vi "TDS - Eurotherm.vi"() -> ()   [LabVIEW 2020]
uses:
  Control 2.ctl
  <instrlib>/rga_lv_85/SRSRGA85.llb/SRSRGAo Units Enumeration.ctl
  <instrlib>/rga_lv_85/SRSRGA85.llb/SRSRGAo RefNum.ctl
  <vilib>/Utility/sysdir.llb/System Directory Type.ctl
  <vilib>/Waveform/WDTFileIO.llb/Export Waveforms To Spreadsheet File (1D).vi
  custom-labview-lib-customlibs/customlib.lvlib
panel:
  out "VISA class":refnum<visa-resource-name>
  out "Process Value":sgl format="%.3g"
  in  "Reference Tab":refnum<vi>[](array[refnum])
  out "heat_LastData":dbl[](array[numeric])
  in  "Reconnect":bool
  out "RGA_LastData":sgl[](array[numeric]) format="%.2f"
  out "size(s) 3":i32
  out "HEAT start time":timestamp=timestamp(3621395400.2120705 s since 1904-01-01)
  out "Label.Text":string="D"
  out "Array 2":waveform(dbl)[](array[waveform])
  out "RGA data":waveform(dbl)[](array[waveform])=[{"t0"=timestamp(3621395444.273366 s since 1904-01-01), "dt"=0.25, "Y"=[0.0]}]
  out "output array":sgl[][](array[numeric])=[[8.752041e-08, 0.0, 0.0, 0.0]]
  out "Boolean":T1=TRUE
  out "stopped_loops":bool=TRUE
  in  "Tab Control":enum32{"Main", "XY Graph", "RGA"}(tab)
  in  "Start 1":bool=TRUE
  in  "Clear ALL":bool
  out "Waveform Graph":waveform(dbl)[](graph)
  out "main Graph":T2(graph)
  in  "Start 3":bool=TRUE
  out "XY Graph 2":cluster{dbl[], dbl[]}[](graph)
  in  "START RGA":bool
  out "Loop Time [ms]":u32=251
  in  "stop 3":bool
  in  "Rate (sec)":dbl=0.25 min=0.001
  out "P vs. t":sgl[][](graph)=[[8.752041e-08, 0.0, 0.0, 0.0]]
  in  "Tab Control 2":enum32{"Eurotherm"}(tab)
  out "Process Value":dbl
  in  "Save Data As":bool
  in  "Tab Control 3":enum32{"RGA control", "RGA setting"}(tab)
  out "CEM:":bool
  out "Filament:":bool
  in  "Disconnect":bool
  in  "Connect":bool
  in  "Connection Type:":u16(ring)=1 items=["Ethernet", "Serial"]
  in  "Specifications":T3(array[cluster])=[{"Mass"=2, "Noise Floor"=4, "CEM "=FALSE}] {"Noise Floor" min=0 max=7; "Mass" min=1 max=100}
  in  "Units:":T4
  in  "CEM:":bool
  in  "Filament:":bool
  out "Conected:":bool
  out "Error:":bool
  in  "START RGA  2":bool
  in  "stop 4":bool
  in  "Electron Emission [mA]":sgl=1.0 format="%.2f"
  out "Act. Electron Emission":sgl format="%.2f"
  out "Numeric":i32
  out "error out":errorcluster
  in  "ionizer":bool
  in  "detector":bool
  in  "stop":bool=TRUE
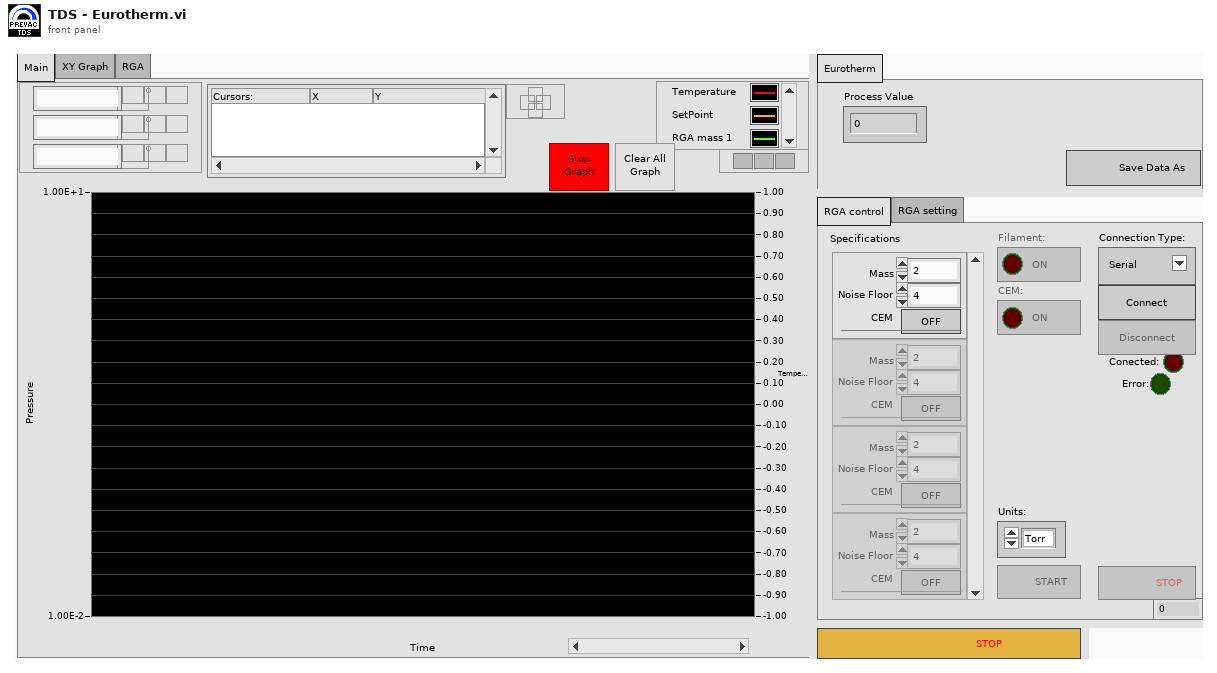
[diagram p1: front panel]
types:
  T1 = typedef "Control 2.ctl" = bool
  T2 = cluster{"heat_LastData[0]":dbl, "heat_LastData[1]":dbl, "heat_LastData[2]":dbl, "heat_LastData[3]":dbl, "heat_LastData[4]":dbl, "heat_LastData[5]":dbl, "heat_LastData[6]":dbl, "heat_LastData[7]":dbl, "heat_LastData[8]":dbl}
  T3 = cluster{"Mass":i32, "Noise Floor":i32, "CEM ":bool}[]
  T4 = typedef "SRSRGAo Units Enumeration.ctl" = enum16{"Torr", "mTorr", "mbar", "bar", "Pa", "A", "ppm"}
  T5 = typedef "SRSRGAo RefNum.ctl" = u16
  T6 = cluster{"heat_LastData[0]":dbl, "heat_LastData[1]":dbl, "heat_LastData[2]":dbl, "heat_LastData[3]":dbl, "heat_LastData[4]":dbl, "heat_LastData[5]":dbl, "heat_LastData[6]":dbl, "heat_LastData[7]":dbl, "heat_LastData[8]":dbl}[]
  T7 = enum8{"Enabled", "Disabled", "Disabled and Grayed Out"}
  T8 = enum16{"Initialize", "Init+Factory", "Init+Fact+Standby"}
  T9 = typedef "LVRectTypeDef.ctl" = cluster{"Left":i16, "Top":i16, "Right":i16, "Bottom":i16}
  T10 = typedef "System Directory Type.ctl" = i32
  T11 = cluster{"Mass":i32, "Noise Floor":i32, "CEM On?":bool}[]
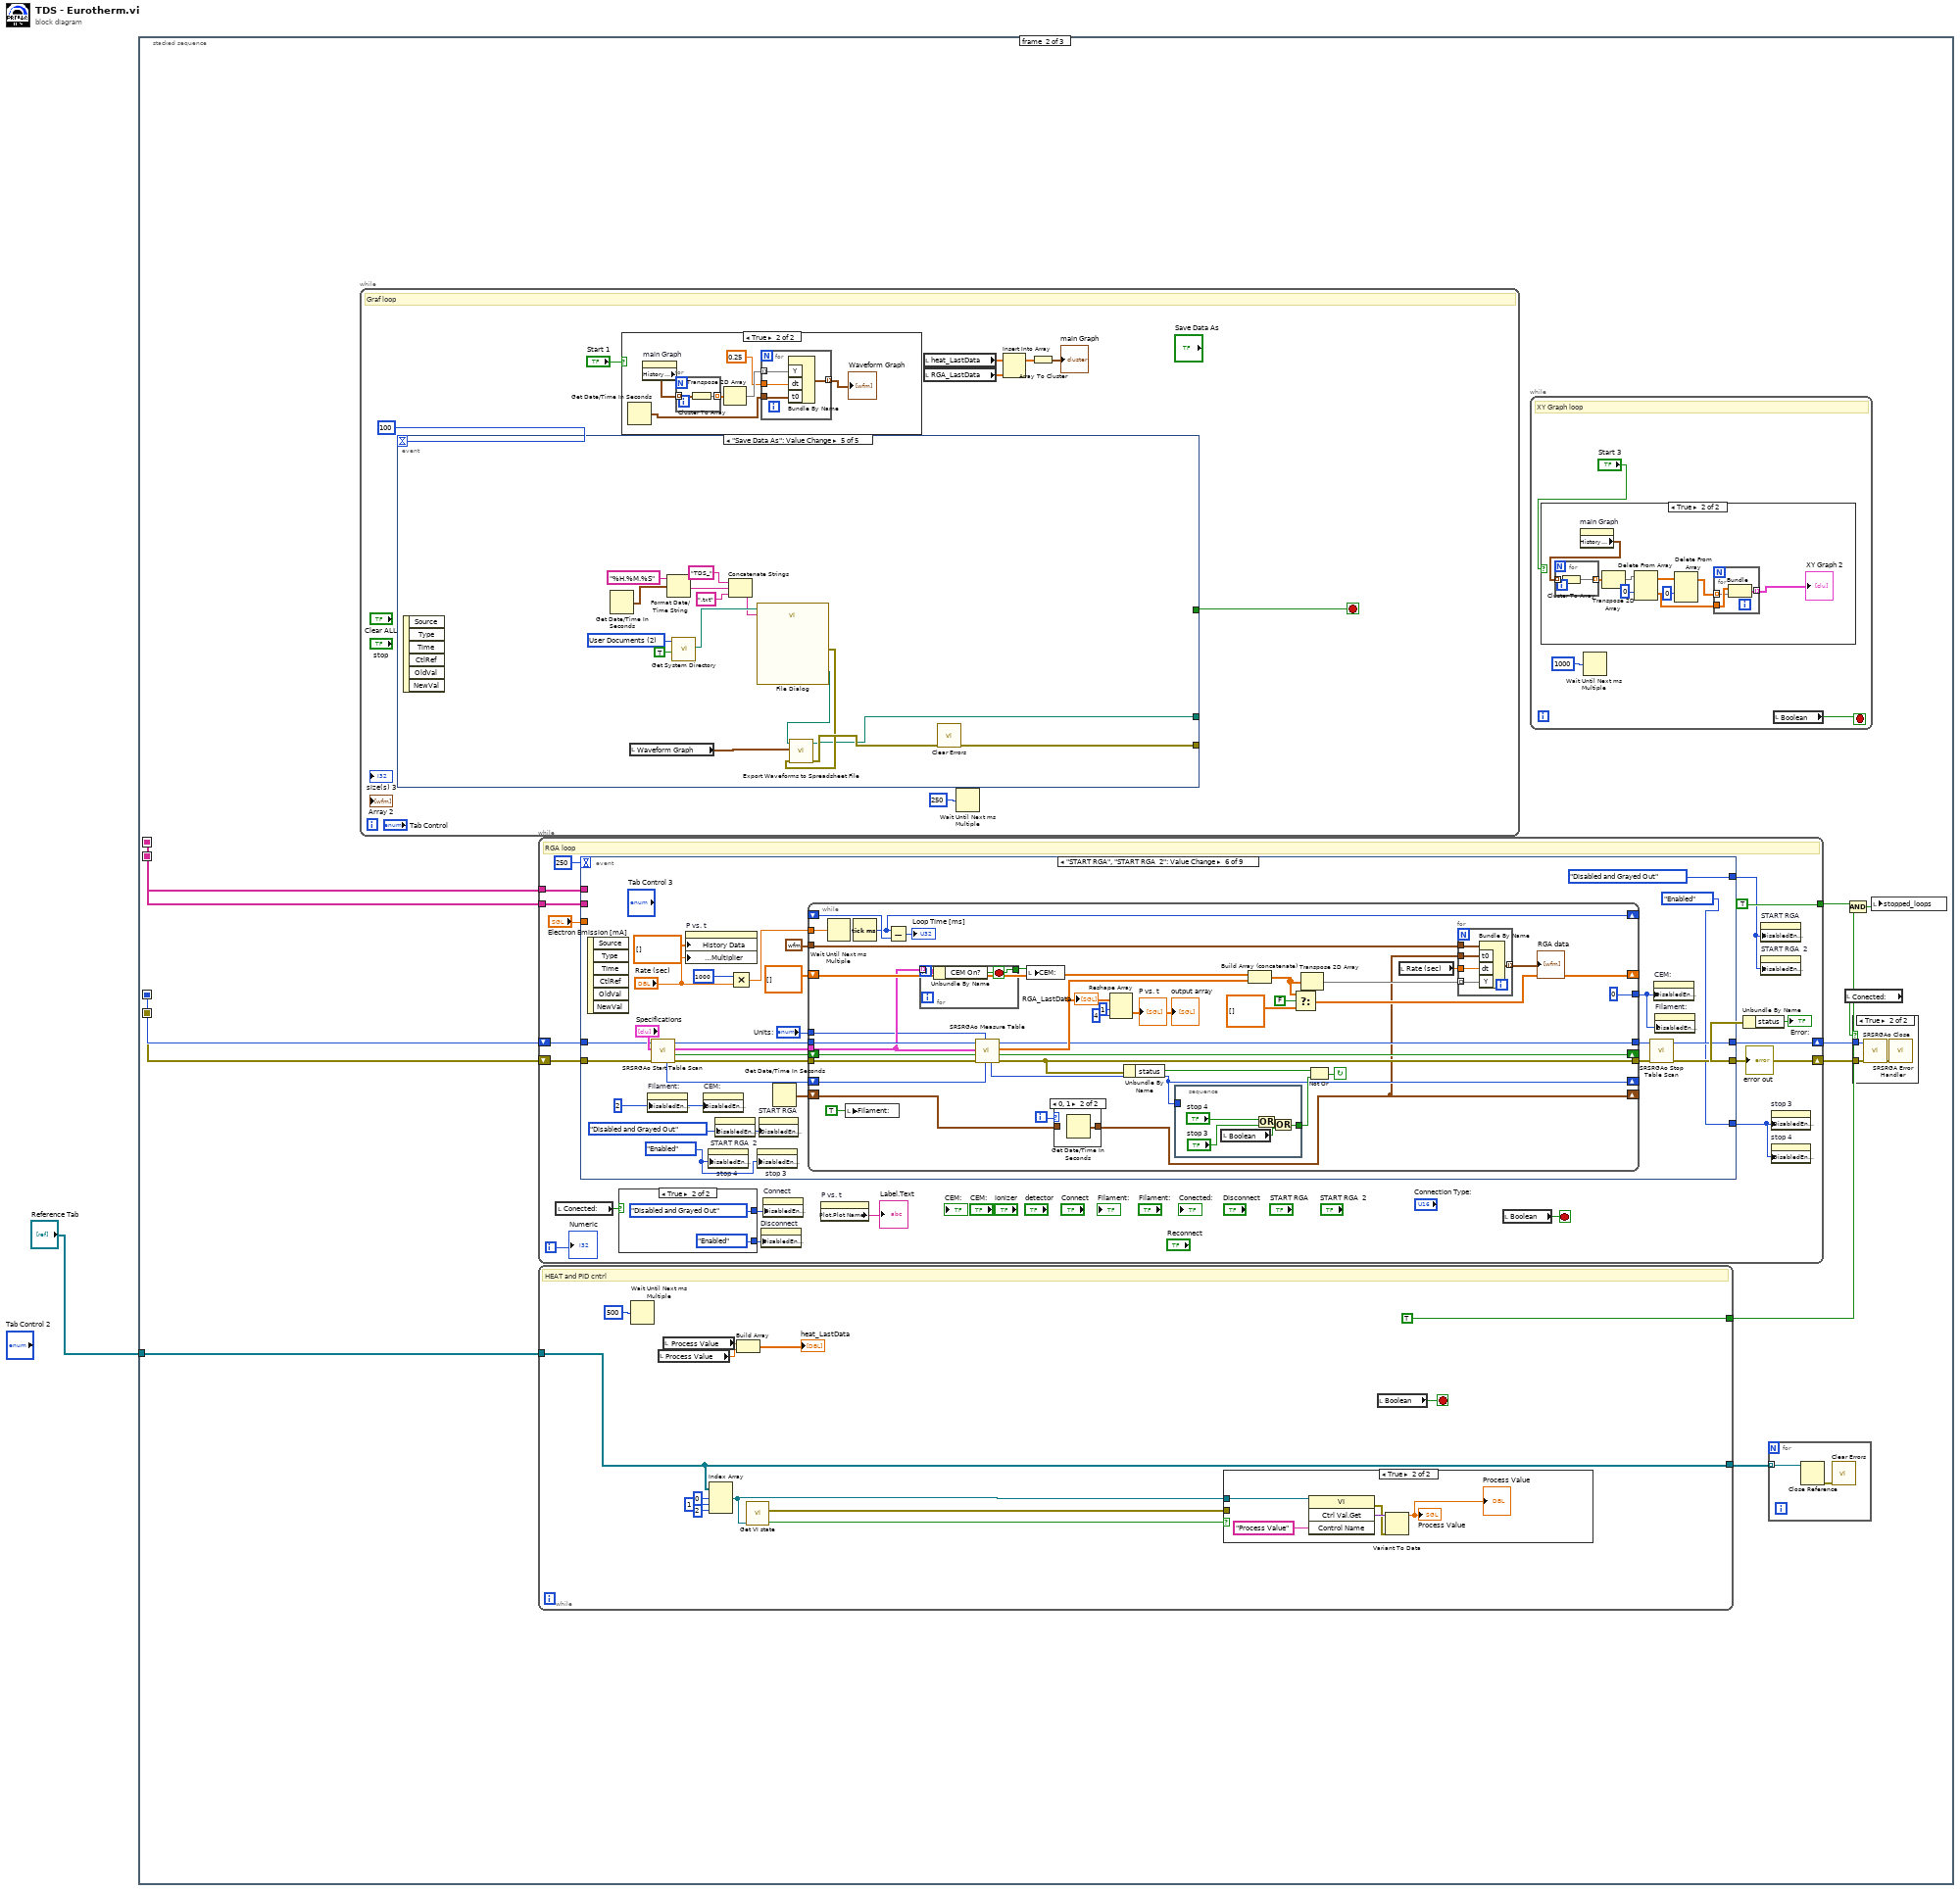
[diagram p0: block diagram]
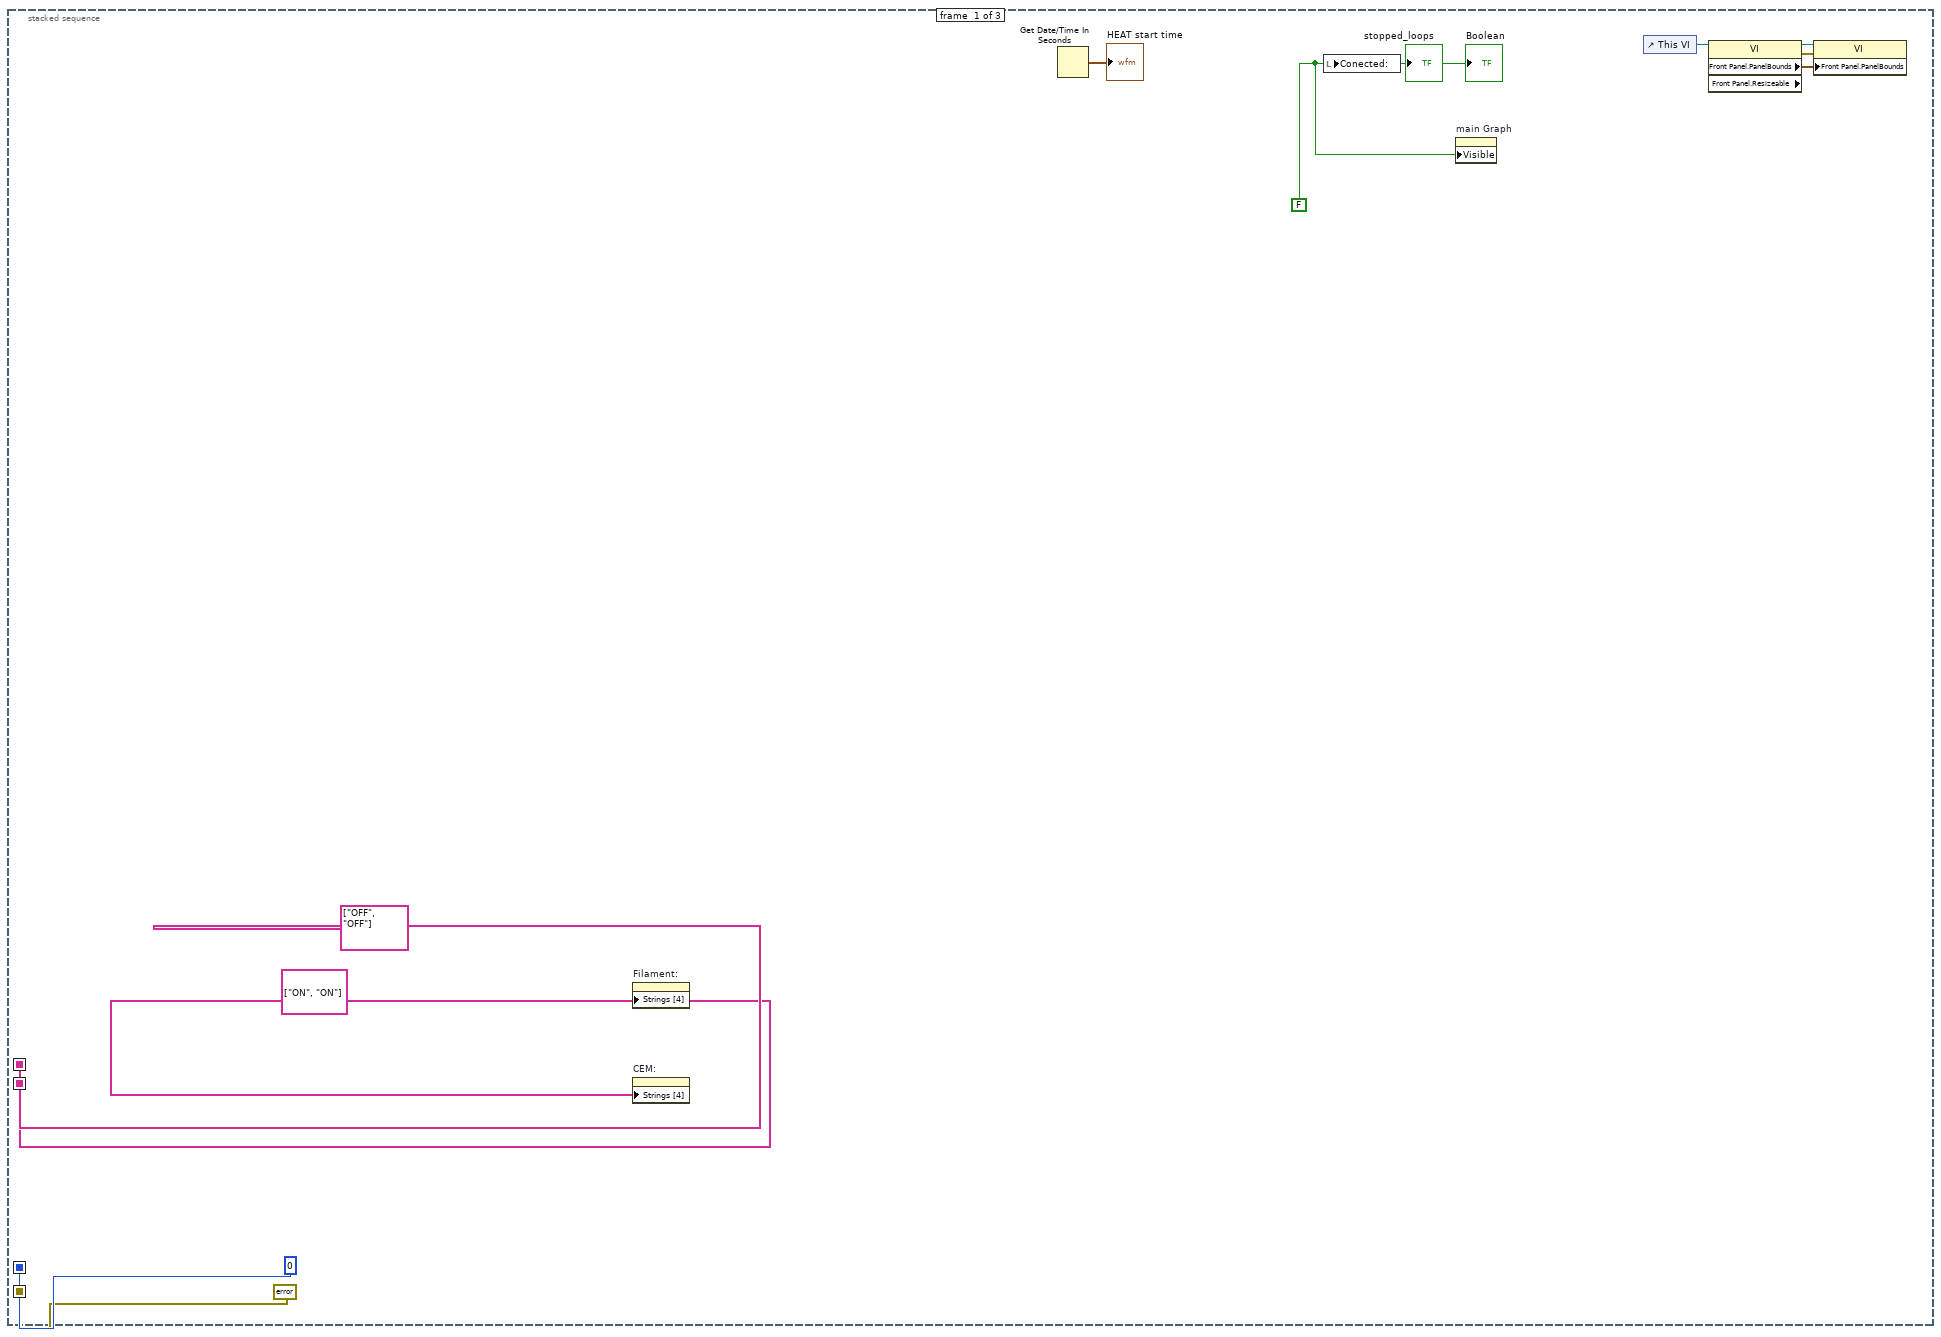
[diagram p2: hidden frame]
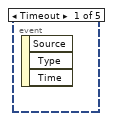
[diagram p7: hidden frame]
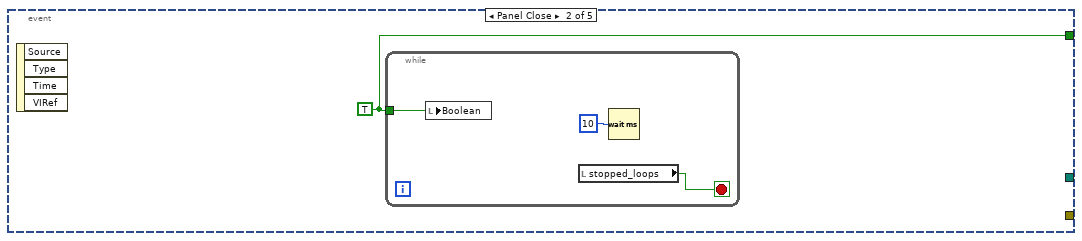
[diagram p8: hidden frame]
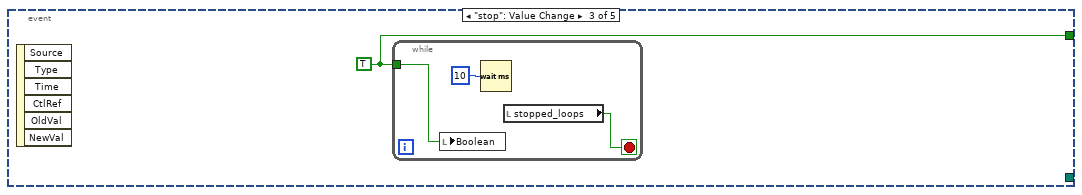
[diagram p9: hidden frame]
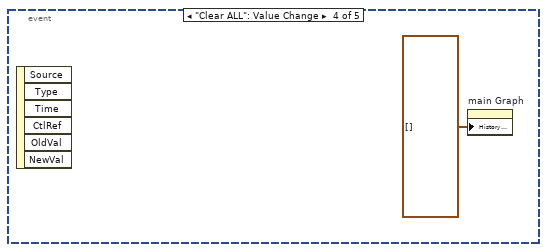
[diagram p10: hidden frame]
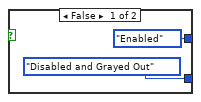
[diagram p11: hidden frame]
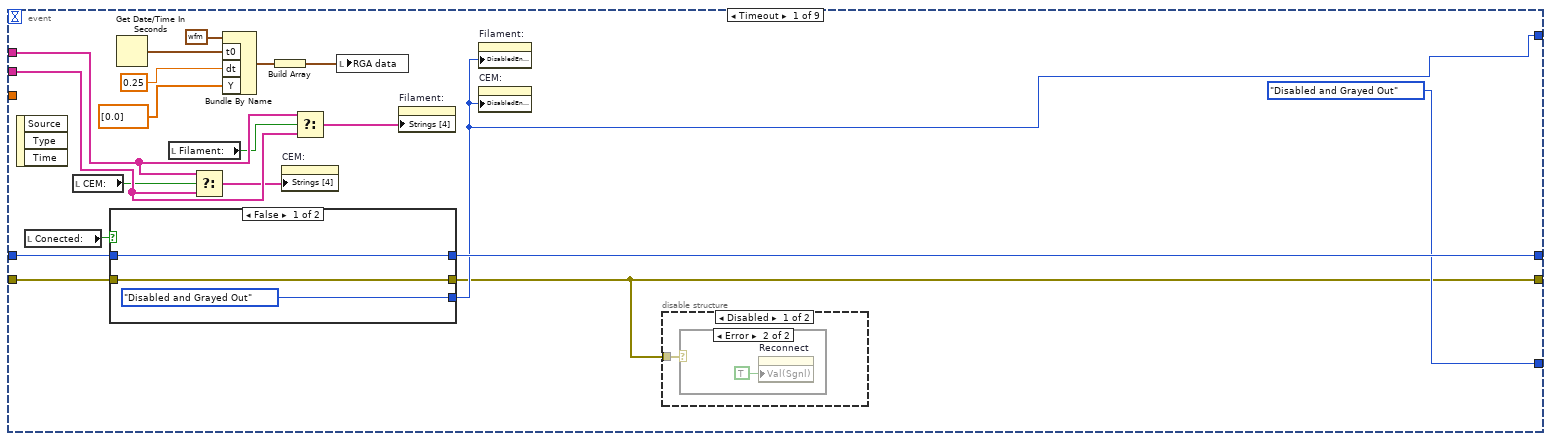
[diagram p12: hidden frame]
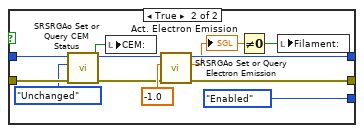
[diagram p15: hidden frame]
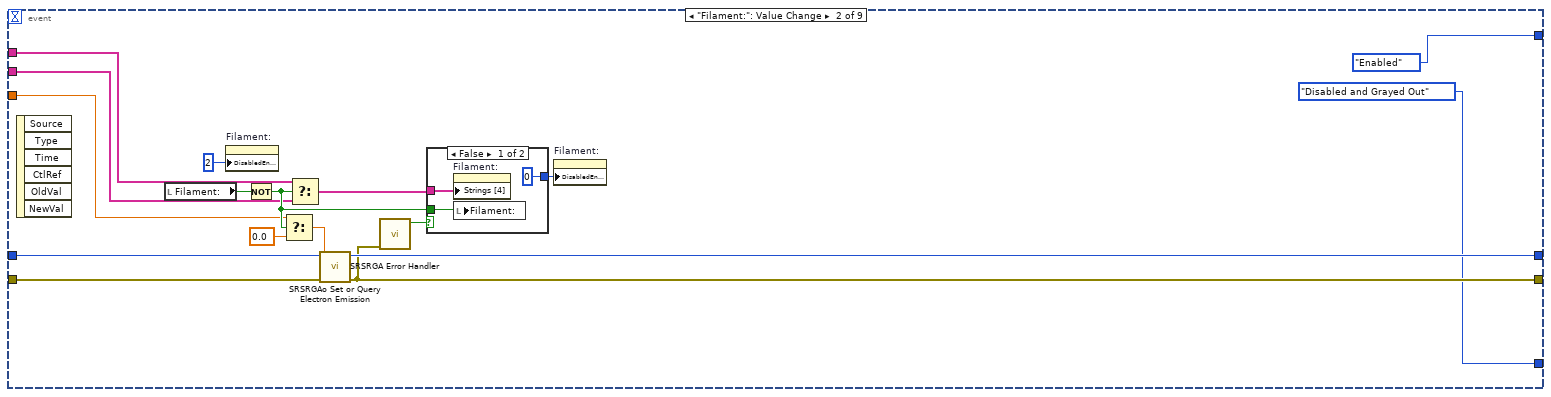
[diagram p16: hidden frame]
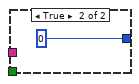
[diagram p17: hidden frame]
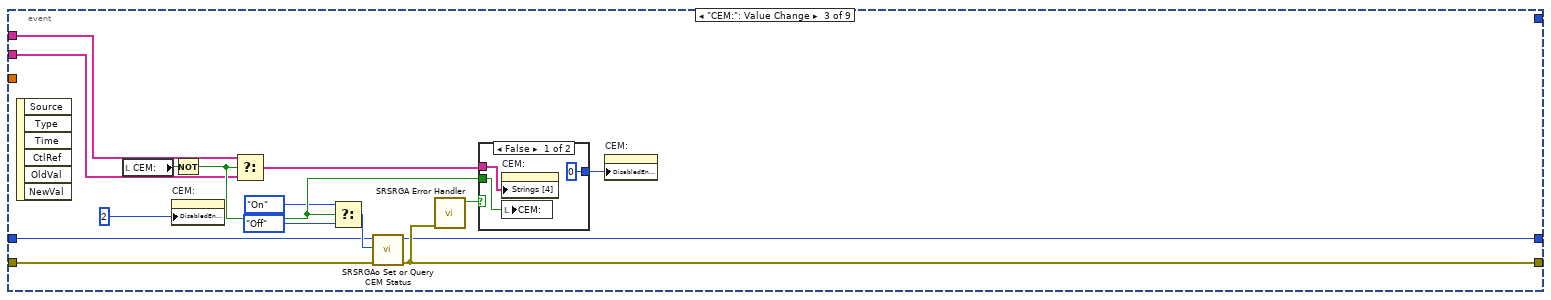
[diagram p18: hidden frame]
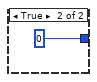
[diagram p19: hidden frame]
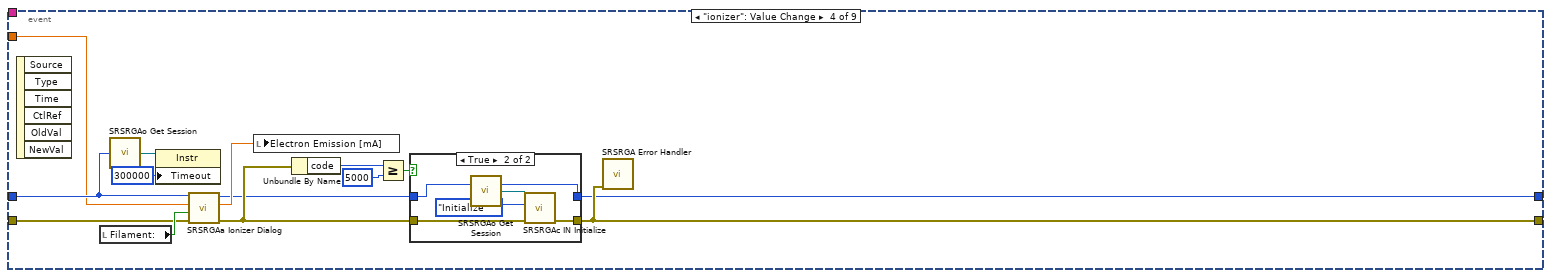
[diagram p20: hidden frame]
diagram:
  n1 = stacked-sequence {
    seq-local: [string[] ["OFF", "OFF"] ("Write Attribute") _ _] -> [_ w20 _]
    seq-local: [w9 _ _] -> [_ w19 _]
    seq-local: [T5 0 ("SRSRGA Refnum") _ _] -> [_ w15 _]
    seq-local: [errorcluster {"status"=FALSE, "code"=0, "source"=""} ("error out") _ _] -> [_ w14 _]
    tunnel: "Reference Tab" -> [_ w13 _]
    frame #0 {
      w9 = string[] ["ON", "ON"] ("Write Attribute")
      w2 = FALSE ("Boolean")
      n2 = property on="Filament:" class="Bool"("Strings [4]"=w9) -> ()  [unwired: 2 in, 2 out]
      n3 = property on="CEM:" class="Bool"("Strings [4]"=w9) -> ()  [unwired: 2 in, 2 out]
      n4 = Get Date/Time In Seconds() -> (seconds since 1Jan1904=→"HEAT start time":timestamp)
      n5 = local write "Conected:"(w2) -> ()
      n6 = property on="main Graph" class="WFChart (strict)"("Visible"=w2) -> ()  [unwired: 2 in, 2 out]
      n7 = control-ref of="This VI"() -> (w8:refnum<vi>)
      n8 = property class="VI" props=["Front Panel.PanelBounds", "Front Panel.Resizeable"](reference=w8) -> (reference out=w6:refnum<vi>, error out=w5:errorcluster, "Front Panel.PanelBounds"=w7:T9)  [unwired: 1 in, 1 out]
      n9 = property class="VI"(reference=w6, error in=w5, "Front Panel.PanelBounds"=w7) -> ()  [unwired: 2 out]
      "stopped_loops" <- w2
      "Boolean" <- w2
    }
    frame #1 {
      n10 = while {
        stop <- w70 stop-if-true
        # "Graf loop"
        n11 = event shown="[4] \"Save Data As\": Value Change" {
          selector: _ -> [_ _ _ _ _]
          dyn-events: _ -> [_ _ _ _ _]
          timeout: 100 -> [_ _ _ _ _]
          tunnel: [_ w84 w88 _ _] -> w70
          tunnel: [_ _ _ _ w95] -> _
          tunnel: [_ _ _ _ w94] -> _
          event Timeout {
            n12 = event-data() -> ()  [unwired: 1 in, 3 out]
          }
          event Panel Close {
            w84 = TRUE
            n13 = event-data() -> ()  [unwired: 1 in, 4 out]
            n14 = while {
              tunnel: w84 -> [w86]
              stop <- w87 stop-if-true
              n15 = local write "Boolean"(w86) -> ()
              n16 = local read "stopped_loops"() -> (w87:bool)
              n17 = Wait (ms)(milliseconds to wait=10) -> ()  [unwired: 1 out]
            }
          }
          event "stop": Value Change {
            w88 = TRUE
            n18 = event-data() -> ()  [unwired: 1 in, 6 out]
            n19 = while {
              tunnel: w88 -> [w89]
              stop <- w91 stop-if-true
              n20 = local write "Boolean"(w89) -> ()
              n21 = Wait (ms)(milliseconds to wait=10) -> ()  [unwired: 1 out]
              n22 = local read "stopped_loops"() -> (w91:bool)
            }
          }
          event "Clear ALL": Value Change {
            n23 = event-data() -> ()  [unwired: 1 in, 6 out]
            n24 = property on="main Graph" class="WFChart (strict)"("History Data"=T6 []) -> ()  [unwired: 2 in, 2 out]
          }
          event "Save Data As": Value Change {
            w106 = T10 2 items=["User Home"=0, "User Desktop"=1, "User Documents"=2, "User Application Data"=3, "User Preferences"=4, "User Temporary"=5, "Public Documents"=6, "Public Application Data"=7, "Public Preferences"=8, "Public Cache"=13, "System Core Libraries"=9, "System Installed Libraries"=10, "Application Files"=11, "Boot Volume Root"=12] ("system directory type")
            n25 = event-data() -> ()  [unwired: 1 in, 6 out]
            n26 = Get Date/Time In Seconds() -> (seconds since 1Jan1904=w104:timestamp)
            n27 = local read "Waveform Graph"() -> (w98:waveform(dbl)[])
            n28 = Format Date/Time String(time format string (%c)="%H.%M.%S", seconds (now)=w104) -> (date/time string=w103:string)  [unwired: 1 in]
            n29 = call <vilib>:"Get System Directory.vi"("create directory if not found? (F)"=TRUE, "system directory type"=w106) -> ("system directory"=w105:path)  [unwired: 9 in]
            n30 = Concatenate Strings("TDS_" ("default name"), w103, ".txt" ("default name")) -> (w101:string)
            n31 = call "File Dialog"("start path"=w105, "default name"=w101) -> ("selected path"=w99:path, "error out"=w96:errorcluster)  [unwired: 10 in, 2 out]
            n32 = call-poly <vilib>:"Export Waveforms to Spreadsheet File.vi"("error in (no error)"=w96, "waveforms"=w98, "file path (dialog if empty)"=w99) -> ("error out"=w100:errorcluster, "new file path (Not A Path if cancelled)"=w95:path)  [unwired: 7 in]
            n33 = call <vilib>:"Clear Errors.vi"("error in (no error)"=w100) -> ("error out"=w94:errorcluster)  [unwired: 5 in, 1 out]
          }
        }
        n34 = case shown="True" "Start 1" {
          frame False {
          }
          frame True {
            n35 = Get Date/Time In Seconds() -> (seconds since 1Jan1904=w74:timestamp)
            n36 = property on="main Graph" class="WFChart (strict)"() -> ("History Data"=w77:T6)  [unwired: 2 in, 2 out]
            n37 = for {
              tunnel: w77 -> [w83] mode=indexing
              tunnel: [w82] -> w76 mode=indexing
              n38 = Cluster To Array(cluster=w83) -> (array=w82:dbl[])
            }
            n39 = Transpose 2D Array(2D array=w76) -> (transposed array=w75:dbl[][])
            n40 = for {
              tunnel: w74 -> [w81]
              tunnel: 0.25 ("y") -> [w80]
              tunnel: w75 -> [w79] mode=indexing
              tunnel: [w78] -> w72 mode=indexing
              n41 = Bundle By Name("Y"=w79, "dt"=w80, "t0"=w81) -> (w78:waveform(dbl))  [unwired: 1 out]
            }
            "Waveform Graph" <- w72
          }
        }
        n42 = local read "heat_LastData"() -> (w65:dbl[])
        n43 = local read "RGA_LastData"() -> (w66:sgl[])
        n44 = Wait Until Next ms Multiple(millisecond multiple=u32 250) -> ()  [unwired: 1 out]
        n45 = Insert Into Array(array=w65, new element=w66) -> (w67:dbl[])  [unwired: 1 in]
        n46 = Array To Cluster(array=w67) -> (cluster=→"main Graph":T2)
      }
      n47 = while {
        tunnel: [TRUE] -> w17
        tunnel: w13 -> [w46]
        tunnel: [w46] -> w12
        stop <- w58 stop-if-true
        # "HEAT and PID cntrl"
        n48 = Wait Until Next ms Multiple(millisecond multiple=u32 500) -> ()  [unwired: 1 out]
        n49 = local read "Process Value"() -> (w54:sgl)
        n50 = local read "Process Value"() -> (w55:sgl)
        n51 = Index Array(array=w46, index #1=0 ("index"), index #2=1 ("index"), index #3=2 ("index")) -> (element #1=w49:refnum<vi>)  [unwired: 2 out]
        n52 = Build Array(w55, w54) -> (→"heat_LastData":sgl[])
        n53 = call "Get VI state.vi"("reference"=w49) -> ("VI is active"=w48:bool, "error out"=w47:errorcluster)  [unwired: 8 in, 1 out]
        n54 = case shown="True" w48 {
          tunnel: w49 -> [_ w61]
          tunnel: w47 -> [_ _]
          frame False {
          }
          frame True {
            n55 = invoke class="VI" method="Ctrl Val.Get"(reference=w61, "Control Name"="Process Value") -> (error out=w60:errorcluster, "Get Control Value Variant"=w62:variant)  [unwired: 2 in, 2 out]
            n56 = Variant To Data(error in=w60, Variant=w62) -> (data=→"Process Value" →"Process Value":sgl)  [unwired: 1 in, 1 out]
          }
        }
        n57 = local read "Boolean"() -> (w58:T1)
      }
      n58 = while {
        tunnel: [TRUE] -> w16
        shift-right: [w125] -> w22
        shift-left: w15 -> [w124]
        shift-right: [w112] -> w21
        shift-left: w14 -> [w123]
        tunnel: w20 -> [w118]
        tunnel: w19 -> [w117]
        i -> [w108]
        stop <- w122 stop-if-true
        # "RGA loop"
        n59 = local read "Conected:"() -> (w115:bool)
        n60 = event shown="[5] \"START RGA\", \"START RGA  2\": Value Change" {
          selector: _ -> [_ _ _ _ _ _ _ _ _]
          dyn-events: _ -> [_ _ _ _ _ _ _ _ _]
          timeout: 250 -> [_ _ _ _ _ _ _ _ _]
          tunnel: [w141 w175 w192 w206 w227 w258 w326 w336 T5 0 ("SRSRGA Refnum")] -> w125
          tunnel: w124 -> [w142 w177 w195 w212 w232 w260 _ w333 w345]
          tunnel: w123 -> [w140 w176 w194 w211 w231 w259 _ w332 w344]
          tunnel: [w130 w174 w193 w210 w230 w257 w325 w335 w342] -> w112
          tunnel: w118 -> [w138 w172 w190 _ _ _ _ _ _]
          tunnel: w117 -> [w137 w171 w189 _ _ _ _ _ _]
          tunnel: "Electron Emission [mA]" -> [_ w168 _ w209 _ _ _ _ _]
          tunnel: [w131 T7."Enabled" ("Disabled") _ _ _ T7."Disabled and Grayed Out" ("Disabled") _ _ _] -> w110
          tunnel: [T7."Disabled and Grayed Out" ("Disabled") T7."Disabled and Grayed Out" ("Disabled") _ _ _ T7."Enabled" ("Disabled") _ _ _] -> w109
          event Timeout {
            n61 = event-data() -> ()  [unwired: 1 in, 3 out]
            n62 = local read "Conected:"() -> (w139:bool)
            n63 = local read "CEM:"() -> (w134:bool)
            n64 = case shown="False" w139 {
              tunnel: w142 -> [w153 w156]
              tunnel: [w153 w164] -> w141
              tunnel: w140 -> [w151 w161]
              tunnel: [w151 w154] -> w130
              tunnel: [T7."Disabled and Grayed Out" ("Disabled") T7."Enabled" ("Disabled")] -> w131
              frame False {
              }
              frame True {
                n65 = call <instrlib>:"SRSRGAo Set or Query CEM Status.vi"("error in (no error)"=w161, "CEM (Unchanged)"=enum16{"Unchanged", "Off", "On"}."Unchanged", "SRSRGA Refnum"=w156) -> ("error out"=w155:errorcluster, "CEM On?"=w159:bool, "SRSRGA Refnum"=w162:T5)  [unwired: 6 in]
                n66 = local write "CEM:"(w159) -> ()
                n67 = call <instrlib>:"SRSRGAo Set or Query Electron Emission.vi"("error in (no error)"=w155, "Electron Emission (1.00 mA)"=sgl -1.0, "SRSRGA Refnum"=w162) -> ("error out"=w154:errorcluster, "Electron Emission"=w158:sgl, "SRSRGA Refnum"=w164:T5)  [unwired: 6 in]
                "Act. Electron Emission" <- w158
                n68 = Not Equal To 0?(x=w158) -> (x != 0?=w163:bool)
                n69 = local write "Filament:"(w163) -> ()
              }
            }
            n70 = Get Date/Time In Seconds() -> (seconds since 1Jan1904=w148:timestamp)
            n71 = local read "Filament:"() -> (w136:bool)
            n72 = Select(t=w138, s=w134, f=w137) -> (s? t:f=w133:string[])
            n73 = Bundle By Name(cluster=waveform(dbl) {"t0"=timestamp(0 s since 1904-01-01), "dt"=1.0, "Y"=[]} ("waveform"), "t0"=w148, "dt"=0.25, "Y"=dbl[] [0.0]) -> (w144:waveform(dbl))
            n74 = Build Array(w144) -> (w143:waveform(dbl)[])
            n75 = property on="CEM:" class="Bool"("Strings [4]"=w133) -> ()  [unwired: 2 in, 2 out]
            n76 = Select(t=w138, s=w136, f=w137) -> (s? t:f=w135:string[])
            n77 = local write "RGA data"(w143) -> ()
            n78 = property on="Filament:" class="Bool"("Strings [4]"=w135) -> ()  [unwired: 2 in, 2 out]
            n79 = property on="Filament:" class="Bool"("DisabledEnum"=w131) -> ()  [unwired: 2 in, 2 out]
            n80 = property on="CEM:" class="Bool"("DisabledEnum"=w131) -> ()  [unwired: 2 in, 2 out]
            n81 = disable-structure shown="Disabled" {
              disable-tunnel: w130 -> [w149 _]
              frame Disabled {
                n82 = case shown="Error" w149 {
                  frame No Error {
                  }
                  frame Error {
                    n83 = property on="Reconnect" class="Bool (strict)"("Val(Sgnl)"=TRUE ("Value (Signaling)")) -> ()  [unwired: 2 in, 2 out]
                  }
                }
              }
              frame Enabled {
              }
            }
          }
          event "Filament:": Value Change {
            n84 = event-data() -> ()  [unwired: 1 in, 6 out]
            n85 = local read "Filament:"() -> (w173:bool)
            n86 = property on="Filament:" class="Bool"("DisabledEnum"=u8 2 ("Write Attribute")) -> ()  [unwired: 2 in, 2 out]
            n87 = Not(x=w173) -> (.not. x?=w179:bool)
            n88 = Select(t=w168, s=w179, f=sgl 0.0) -> (s? t:f=w182:sgl)
            n89 = Select(t=w172, s=w179, f=w171) -> (s? t:f=w178:string[])
            n90 = call <instrlib>:"SRSRGAo Set or Query Electron Emission.vi"("error in (no error)"=w176, "Electron Emission (1.00 mA)"=w182, "SRSRGA Refnum"=w177) -> ("error out"=w174:errorcluster, "SRSRGA Refnum"=w175:T5)  [unwired: 6 in, 1 out]
            n91 = call <instrlib>:"SRSRGA Error Handler.vi"("error in (no error)"=w174) -> ("error?"=w180:bool)  [unwired: 9 in, 1 out]
            n92 = case shown="False" w180 {
              tunnel: w179 -> [w184 _]
              tunnel: [u8 0 ("Write Attribute") u8 0 ("Write Attribute")] -> w169
              tunnel: w178 -> [w183 _]
              frame False {
                n93 = property on="Filament:" class="Bool"("Strings [4]"=w183) -> ()  [unwired: 2 in, 2 out]
                n94 = local write "Filament:"(w184) -> ()
              }
              frame True {
              }
            }
            n95 = property on="Filament:" class="Bool"("DisabledEnum"=w169) -> ()  [unwired: 2 in, 2 out]
          }
          event "CEM:": Value Change {
            n96 = event-data() -> ()  [unwired: 1 in, 6 out]
            n97 = local read "CEM:"() -> (w191:bool)
            n98 = property on="CEM:" class="Bool"("DisabledEnum"=u8 2 ("Write Attribute")) -> ()  [unwired: 2 in, 2 out]
            n99 = Not(x=w191) -> (.not. x?=w199:bool)
            n100 = Select(t=w190, s=w199, f=w189) -> (s? t:f=w200:string[])
            n101 = Select(t=enum16{"Unchanged", "Off", "On"}."On" ("CEM (Unchanged)"), s=w199, f=enum16{"Unchanged", "Off", "On"}."Off" ("CEM (Unchanged)")) -> (s? t:f=w198:enum16{"Unchanged", "Off", "On"})
            n102 = call <instrlib>:"SRSRGAo Set or Query CEM Status.vi"("error in (no error)"=w194, "CEM (Unchanged)"=w198, "SRSRGA Refnum"=w195) -> ("error out"=w193:errorcluster, "SRSRGA Refnum"=w192:T5)  [unwired: 6 in, 1 out]
            n103 = call <instrlib>:"SRSRGA Error Handler.vi"("error in (no error)"=w193) -> ("error?"=w201:bool)  [unwired: 9 in, 1 out]
            n104 = case shown="False" w201 {
              tunnel: w199 -> [w202 _]
              tunnel: [u8 0 ("Write Attribute") u8 0 ("Write Attribute")] -> w187
              tunnel: w200 -> [w203 _]
              frame False {
                n105 = property on="CEM:" class="Bool"("Strings [4]"=w203) -> ()  [unwired: 2 in, 2 out]
                n106 = local write "CEM:"(w202) -> ()
              }
              frame True {
              }
            }
            n107 = property on="CEM:" class="Bool"("DisabledEnum"=w187) -> ()  [unwired: 2 in, 2 out]
          }
          event "ionizer": Value Change {
            n108 = event-data() -> ()  [unwired: 1 in, 6 out]
            n109 = local read "Filament:"() -> (w213:bool)
            n110 = call <instrlib>:"SRSRGAo Get Session.vi"("SRSRGA Refnum"=w212) -> ("SRSRGA Session"=w215:refnum<visa-resource-name>)
            n111 = property class="Instr"(reference=w215, "Timeout"=u32 300000 ("General Settings:Timeout Value")) -> ()  [unwired: 1 in, 2 out]
            n112 = call <instrlib>:"SRSRGAa Ionizer Dialog.vi"("error in (no error)"=w211, "Emission On?"=w213, "Electron Emission (0.02-3.50 mA)"=w209, "SRSRGA Refnum"=w212) -> ("error out"=w216:errorcluster, "Electron Emission"=w208:sgl, "SRSRGA Refnum"=w207:T5)  [unwired: 5 in]
            n113 = local write "Electron Emission [mA]"(w208) -> ()
            n114 = Unbundle By Name(w216) -> ("code"=w219:i32)
            n115 = Greater Or Equal?(x=w219, y=5000) -> (x >= y?=w217:bool)
            n116 = case shown="True" w217 {
              tunnel: w216 -> [w221 w225]
              tunnel: [w221 w224] -> w210
              tunnel: w207 -> [w220 w222]
              tunnel: [w220 w222] -> w206
              frame False {
              }
              frame True {
                n117 = call <instrlib>:"SRSRGAo Get Session.vi"("SRSRGA Refnum"=w222) -> ("SRSRGA Session"=w223:refnum<visa-resource-name>)
                n118 = call <instrlib>:"SRSRGAc IN Initialize.vi"("error in (no error)"=w225, "Initialization Level"=T8."Initialize", "SRSRGA Session"=w223) -> ("error out"=w224:errorcluster)  [unwired: 5 in, 3 out]
              }
            }
            n119 = call <instrlib>:"SRSRGA Error Handler.vi"("error in (no error)"=w210) -> ()  [unwired: 9 in, 2 out]
          }
          event "detector": Value Change {
            n120 = event-data() -> ()  [unwired: 1 in, 6 out]
            n121 = call <instrlib>:"SRSRGAo Get Session.vi"("SRSRGA Refnum"=w232) -> ("SRSRGA Session"=w234:refnum<visa-resource-name>)
            n122 = property class="Instr"(reference=w234, "Timeout"=u32 300000 ("General Settings:Timeout Value")) -> ()  [unwired: 1 in, 2 out]
            n123 = local read "CEM:"() -> (w229:bool)
            n124 = call <instrlib>:"SRSRGAa Detector Dialog.vi"("error in (no error)"=w231, "CEM On?"=w229, "SRSRGA Refnum"=w232) -> ("error out"=w235:errorcluster, "SRSRGA Refnum"=w228:T5)  [unwired: 7 in]
            n125 = Unbundle By Name(w235) -> ("code"=w238:i32)
            n126 = Greater Or Equal?(x=w238, y=5000) -> (x >= y?=w236:bool)
            n127 = case shown="True" w236 {
              tunnel: w235 -> [w240 w243]
              tunnel: [w240 w242] -> w230
              tunnel: w228 -> [w239 w241]
              tunnel: [w239 w241] -> w227
              frame False {
              }
              frame True {
                n128 = call <instrlib>:"SRSRGAo Get Session.vi"("SRSRGA Refnum"=w241) -> ("SRSRGA Session"=w244:refnum<visa-resource-name>)
                n129 = call <instrlib>:"SRSRGAc IN Initialize.vi"("error in (no error)"=w243, "Initialization Level"=T8."Initialize", "SRSRGA Session"=w244) -> ("error out"=w242:errorcluster)  [unwired: 5 in, 3 out]
              }
            }
            n130 = call <instrlib>:"SRSRGA Error Handler.vi"("error in (no error)"=w230) -> ()  [unwired: 9 in, 2 out]
          }
          event "START RGA", "START RGA  2": Value Change {
            w247 = T7."Disabled and Grayed Out" ("Disabled")
            w246 = T7."Enabled" ("Disabled")
            w251 = u8 2 ("Write Attribute")
            n131 = event-data() -> ()  [unwired: 1 in, 6 out]
            n132 = property on="Filament:" class="Bool"("DisabledEnum"=w251) -> ()  [unwired: 2 in, 2 out]
            n133 = call <instrlib>:"SRSRGAo Start Table Scan.vi"("error in (no error)"=w259, "Specifications"="Specifications", "SRSRGA Refnum"=w260) -> ("error out"=w271:errorcluster, "CEM On?"=w268:bool, "Specifications"=w269:T11, "SRSRGA Refnum"=w270:T5, "Noise Floor"=w267:i32)  [unwired: 4 in]
            n134 = property on="P vs. t" class="WFChart (strict)"("History Data"=sgl[][] [] ("Write Attribute"), "X Scale.Offset and Multiplier:Multiplier"="Rate (sec)") -> ()  [unwired: 2 in, 2 out]
            n135 = property on="CEM:" class="Bool"("DisabledEnum"=w251) -> ()  [unwired: 2 in, 2 out]
            n136 = property on="stop 4" class="Bool"("DisabledEnum"=w246) -> ()  [unwired: 2 in, 2 out]
            n137 = property on="START RGA  2" class="Bool"("DisabledEnum"=w247) -> ()  [unwired: 2 in, 2 out]
            n138 = Multiply(x=1000, y="Rate (sec)") -> (x*y=w263:dbl)
            n139 = property on="stop 3" class="Bool"("DisabledEnum"=w246) -> ()  [unwired: 2 in, 2 out]
            n140 = property on="START RGA" class="Bool"("DisabledEnum"=w247) -> ()  [unwired: 2 in, 2 out]
            n141 = Get Date/Time In Seconds() -> (seconds since 1Jan1904=w253:timestamp)
            n142 = while {
              tunnel: w263 -> [w293]
              tunnel: [w284] -> w256
              tunnel: "Units:" -> [w273]
              shift-left: w267 -> [w303]
              shift-right: [w274] -> _
              tunnel: [w283] -> w255
              shift-left: w268 -> [w305]
              shift-right: [w304] -> _
              tunnel: w269 -> [w281]
              tunnel: w270 -> [w306]
              tunnel: w271 -> [w307]
              shift-right: [w295] -> _
              shift-left: _ -> [w297]
              tunnel: waveform(dbl) {"t0"=timestamp(0 s since 1904-01-01), "dt"=1.0, "Y"=[]} ("waveform") -> [w294]
              shift-right: [w276] -> _
              shift-left: sgl[][] [] -> [w290]
              shift-right: [w272] -> _
              shift-left: w253 -> [w286]
              tunnel: [u8 0 ("Write Attribute")] -> w250
              i -> [w287]
              stop <- w300 continue-if-true
              n143 = Wait Until Next ms Multiple(millisecond multiple=w293) -> ()  [unwired: 1 out]
              n144 = local write "Filament:"(TRUE ("Filament")) -> ()
              n145 = Tick Count (ms)() -> (millisecond timer value=w295:u32)
              n146 = Subtract(x=w295, y=w297) -> (x-y=→"Loop Time [ms]":u32)
              n147 = for {
                tunnel: w281 -> [w309] mode=indexing
                tunnel: [w308] -> w280
                stop <- w308 stop-if-true
                n148 = Unbundle By Name(w309) -> ("CEM On?"=w308:bool)
              }
              n149 = call <instrlib>:"SRSRGAo Measure Table.vi"("Entrance Noise Floor"=w303, "Units"=w273, "error in (no error)"=w307, "Entrance CEM On?"=w305, "Specifications"=w281, "SRSRGA Refnum"=w306) -> ("error out"=w283:errorcluster, "Exit CEM On?"=w304:bool, "Readings in Units"=w285:sgl[], "SRSRGA Refnum"=w284:T5, "Exit Noise Floor"=w274:i32)  [unwired: 1 in]
              "RGA_LastData" <- w285
              n150 = local write "CEM:"(w280) -> ()
              n151 = case shown="0, 1" w287 {
                tunnel: [w310 w311] -> w272
                tunnel: w286 -> [w310 _]
                frame 2, Default {
                }
                frame 0, 1 {
                  n152 = Get Date/Time In Seconds() -> (seconds since 1Jan1904=w311:timestamp)
                }
              }
              n153 = Reshape Array(w285, 1 ("Dimension Size"), 4 ("Dimension Size")) -> (→"P vs. t" →"output array":sgl[][])
              n154 = Unbundle By Name(w283) -> ("status"=w302:bool)
              n155 = stacked-sequence {
                tunnel: [w321] -> w301
                tunnel: w274 -> [_]
                frame #0 {
                  n156 = local read "Boolean"() -> (w320:T1)
                  n157 = Or(x="stop 4", y="stop 3") -> (x .or. y?=w317:bool)
                  n158 = Or(x=w317, y=w320) -> (x .or. y?=w321:T1)
                }
              }
              n159 = Build Array (concatenate)(w290, w285) -> (w278:dbl[][])
              n160 = Select(t=w278, s=FALSE ("build array of data?"), f=dbl[][] []) -> (s? t:f=w276:dbl[][])
              n161 = Transpose 2D Array(2D array=w278) -> (transposed array=w289:dbl[][])
              n162 = Not Or(1:w301, 2:w302) -> (0:w300:T1)
              n163 = local read "Rate (sec)"() -> (w288:dbl)
              n164 = for {
                tunnel: w272 -> [w316]
                tunnel: w289 -> [w314] mode=indexing
                tunnel: w294 -> [w315]
                tunnel: w288 -> [w313]
                tunnel: [w312] -> w292 mode=indexing
                n165 = Bundle By Name(cluster=w315, "t0"=w316, "dt"=w313, "Y"=w314) -> (w312:waveform(dbl))
              }
              "RGA data" <- w292
            }
            n166 = call <instrlib>:"SRSRGAo Stop Table Scan.vi"("error in (no error)"=w255, "SRSRGA Refnum"=w256) -> ("error out"=w257:errorcluster, "SRSRGA Refnum"=w258:T5)  [unwired: 8 in]
            n167 = property on="CEM:" class="Bool"("DisabledEnum"=w250) -> ()  [unwired: 2 in, 2 out]
            n168 = property on="Filament:" class="Bool"("DisabledEnum"=w250) -> ()  [unwired: 2 in, 2 out]
          }
          event "Connect": Value Change {
            n169 = event-data() -> ()  [unwired: 1 in, 6 out]
            n170 = local read "Connection Type:"() -> (w327:u16)
            n171 = call <instrlib>:"SRSRGAo Open.vi"("Reinitialize? (True)"=TRUE ("Reinitialize? (False)"), "Connection Type"=w327) -> ("error out"=w325:errorcluster, "SRSRGA Refnum"=w326:T5, "VISA class"=→"VISA class":refnum<visa-resource-name>)  [unwired: 3 in, 4 out]
            n172 = case shown="Error" w325 {
              tunnel: [TRUE FALSE] -> w324
              frame No Error {
              }
              frame Error {
              }
            }
            n173 = local write "Conected:"(w324) -> ()
            n174 = local write "Reconnect"(FALSE ("Reconnect")) -> ()
          }
          event "Reconnect": Value Change {
            n175 = event-data() -> ()  [unwired: 1 in, 6 out]
            n176 = call <instrlib>:"SRSRGAo Close.vi"("error in (no error)"=w332, "SRSRGA Refnum"=w333) -> ()  [unwired: 9 in, 1 out]
            n177 = local read "Connection Type:"() -> (w337:u16)
            n178 = call <instrlib>:"SRSRGAo Open.vi"("Reinitialize? (True)"=TRUE ("Reinitialize? (False)"), "Connection Type"=w337) -> ("error out"=w335:errorcluster, "SRSRGA Refnum"=w336:T5)  [unwired: 3 in, 5 out]
            n179 = case shown="Error" w335 {
              tunnel: [TRUE FALSE] -> w334
              frame No Error {
              }
              frame Error {
              }
            }
            n180 = local write "Conected:"(w334) -> ()
            n181 = local write "Reconnect"(FALSE ("Reconnect")) -> ()
          }
          event "Disconnect": Value Change {
            n182 = event-data() -> ()  [unwired: 1 in, 6 out]
            n183 = call <instrlib>:"SRSRGAo Close.vi"("error in (no error)"=w344, "SRSRGA Refnum"=w345) -> ("error out"=w342:errorcluster)  [unwired: 9 in]
            n184 = local write "Conected:"(FALSE) -> ()
          }
        }
        "error out" <- w112
        n185 = case shown="True" w115 {
          tunnel: [T7."Enabled" ("Disabled") T7."Disabled and Grayed Out" ("Disabled")] -> w114
          tunnel: [T7."Disabled and Grayed Out" ("Disabled") T7."Enabled" ("Disabled")] -> w113
          frame False {
          }
          frame True {
          }
        }
        n186 = property on="Disconnect" class="Bool"("DisabledEnum"=w113) -> ()  [unwired: 2 in, 2 out]
        n187 = property on="Connect" class="Bool"("DisabledEnum"=w114) -> ()  [unwired: 2 in, 2 out]
        n188 = property on="P vs. t" class="WFChart (strict)"() -> ("Plot.Plot Name"=→"Label.Text":string)  [unwired: 2 in, 2 out]
        n189 = local read "Boolean"() -> (w122:T1)
        n190 = Unbundle By Name(w112) -> ("status"=→"Error:":bool)
        n191 = property on="START RGA" class="Bool"("DisabledEnum"=w110) -> ()  [unwired: 2 in, 2 out]
        n192 = property on="START RGA  2" class="Bool"("DisabledEnum"=w110) -> ()  [unwired: 2 in, 2 out]
        n193 = property on="stop 3" class="Bool"("DisabledEnum"=w109) -> ()  [unwired: 2 in, 2 out]
        n194 = property on="stop 4" class="Bool"("DisabledEnum"=w109) -> ()  [unwired: 2 in, 2 out]
        "Numeric" <- w108
      }
      n195 = while {
        stop <- w28 stop-if-true
        # "XY Graph loop"
        n196 = case shown="True" "Start 3" {
          frame False {
          }
          frame True {
            n197 = property on="main Graph" class="WFChart (strict)"() -> ("History Data"=w31:T6)  [unwired: 2 in, 2 out]
            n198 = for {
              tunnel: w31 -> [w42] mode=indexing
              tunnel: [w41] -> w33 mode=indexing
              n199 = Cluster To Array(cluster=w42) -> (array=w41:dbl[])
            }
            n200 = Transpose 2D Array(2D array=w33) -> (transposed array=w29:dbl[][])
            n201 = Delete From Array(array=w29, index (row)=0) -> (deleted portion=w34:dbl[], array with subset deleted=w36:dbl[][])  [unwired: 2 in]
            n202 = Delete From Array(array=w36, index (row)=0) -> (array with subset deleted=w32:dbl[][])  [unwired: 2 in, 1 out]
            n203 = for {
              tunnel: w32 -> [w39] mode=indexing
              tunnel: w34 -> [w40]
              tunnel: [w38] -> w30 mode=indexing
              n204 = Bundle(w40, w39) -> (w38:cluster{dbl[], dbl[]})  [unwired: 1 in]
            }
            "XY Graph 2" <- w30
          }
        }
        n205 = Wait Until Next ms Multiple(millisecond multiple=u32 1000) -> ()  [unwired: 1 out]
        n206 = local read "Boolean"() -> (w28:T1)
      }
      n207 = for {
        tunnel: w12 -> [w25] mode=indexing
        n208 = Close Reference(reference=w25) -> (error out=w24:errorcluster)  [unwired: 1 in]
        n209 = call <vilib>:"Clear Errors.vi"("error in (no error)"=w24) -> ()  [unwired: 5 in, 2 out]
      }
      n210 = local read "Conected:"() -> (w18:bool)
      n211 = Compound Arithmetic op=AND(w16, w17) -> (w23:bool)
      n212 = case shown="True" w18 {
        tunnel: w22 -> [_ w44]
        tunnel: w21 -> [_ w43]
        frame False {
        }
        frame True {
          n213 = call <instrlib>:"SRSRGAo Close.vi"("error in (no error)"=w43, "SRSRGA Refnum"=w44) -> ("error out"=w45:errorcluster)  [unwired: 9 in]
          n214 = call <instrlib>:"SRSRGA Error Handler.vi"("error in (no error)"=w45) -> ()  [unwired: 9 in, 2 out]
        }
      }
      n215 = local write "stopped_loops"(w23) -> ()
    }
    frame #2 {
    }
  }
